vi "NQ Computer Resources.vi"(8 "error in (no error)":errorcluster) -> (0 "error out":errorcluster)   [LabVIEW 2020]
doc: "This VI gets computer resources available to for computing and enqueues that onto the telemtry handler."
uses:
  Type Definitions/Enum - Metadata.ctl
  Type Definitions/Payload Class.ctl
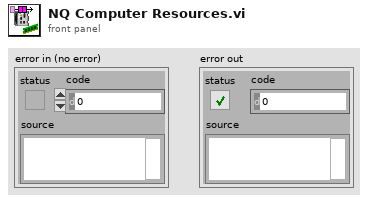
[diagram p1: front panel]
types:
  T1 = typedef "Payload Class.ctl" = enum16{"System State", "Parameters", "Metadata", "Software Monitor", "Data", "Commands"}
  T2 = typedef "Enum - Metadata.ctl" = enum16{"Computer Metadata", "Computer Resources", "RT Image Metadata", "Startup Settings", "Telemetry Recorder Status"}
  T3 = typedef "Computer Resources.ctl" = cluster{"CPU Count":i32, "CPU Speed":u32, "Total Physical Memory":dbl, "Total Virtual Memory":dbl, "Primary Disk Capacity":dbl}
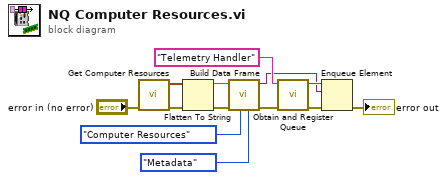
[diagram p0: block diagram]
diagram:
  n1 = call "Get Computer Resources.vi"("error in (no error)"="error in (no error)") -> ("error out"=w11:errorcluster, "Computer Resources"=w10:T3)  [unwired: 9 in]
  n2 = Flatten To String(anything=w10, error in (no error)=w11) -> (data string=w9:string, error out=w6:errorcluster)  [unwired: 2 in, 1 out]
  n3 = call "Build Data Frame.vi"("Payload Class (Data)"=Payload_Class."Metadata", "Payload ID (0)"=Enum_-_Metadata."Computer Resources", "error in (no error)"=w6, "Payload (Empty String)"=w9) -> ("error out"=w2:errorcluster, "Frame"=w3:variant)  [unwired: 6 in]
  n4 = call "Obtain and Register Queue.vi"("error in (no error)"=w2, "name (unnamed)"="Telemetry Handler") -> ("error out"=w1:errorcluster, "Queue Out"=w4:refnum<queue>)  [unwired: 6 in, 2 out]
  n5 = Enqueue Element(queue=w4, element=w3, error in (no error)=w1) -> (error out=→"error out":errorcluster)  [unwired: 1 in, 2 out]
